vi "Encoder Reset.vi"(11 "Name of Encoder":string) -> ()   [LabVIEW 2016]
uses:
  Robot Global Data.vi
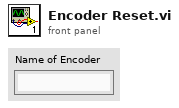
[diagram p1: front panel]
types:
  T1 = typedef "WPI_MotorControlDeviceRef.ctl" = cluster{"DeviceStatus":errorcluster, "Type":T2, "PWM":cluster{"PWM Channel":T3, "DeadBand":T4}, "CAN":cluster{"Device Number":u8, "SetOutput VI Ref":variant, "GetOutput VI Ref":variant, "Enable VI Ref":variant, "Disable VI Ref":variant, "Data":variant}, "Invert":bool}
  T2 = typedef "WPI_MotorControlType.ctl" = enum16{"PWM", "CAN"}
  T3 = typedef "FPGA_DIOPWMChannel.ctl" = enum8{"PWM 0", "PWM 1", "PWM 2", "PWM 3", "PWM 4", "PWM 5", "PWM 6", "PWM 7", "PWM 8", "PWM 9", "PWM MXP 0", "PWM MXP 1", "PWM MXP 2", "PWM MXP 3", "PWM MXP 4", "PWM MXP 5", "PWM MXP 6", "PWM MXP 7", "PWM MXP 8", "PWM MXP 9", "Invalid"}
  T4 = typedef "WPI_PWMDeadband.ctl" = cluster{"Name":string, "maxPositivePwm":i32, "minPositivePwm":i32, "centerPwm":i32, "maxNegativePwm":i32, "minNegativePwm":i32, "angularRange":u16}
  T5 = typedef "WPI_CANTalonSRX_GlobalStatus.ctl" = cluster{"Applied Throttle":dbl, "Module Enabled":bool, "CAN Error":errorcluster, "Closed Loop Error":dbl, "Forward Limit Switch Closed":bool, "Reverse Limit Switch Closed":bool, "Sensor Position":dbl, "Sensor Velocity":dbl, "Current":dbl, "Sticky Fault - Over Temp":bool, "Sticky Fault - Under Voltage":bool, "Sticky Fault - Forward Limit":bool, "Sticky Fault - Reverse Limit":bool, "Sticky Fault - Forward Soft Limit":bool, "Sticky Fault - Reverse Soft Limit":bool, "Brake is Enabled":bool, "Encoder Position":dbl, "Encoder Velocity":dbl, "Encoder Index Count":dbl, "Encoder A Pin State":bool, "Encoder B Pin State":bool, "Encoder Index Pin State":bool, "Analog In":dbl, "Analog In Velocity":dbl, "Temperature (C)":dbl, "Battery Voltage":dbl, "Control 5 Is Supported":bool, "Current Profile Slot Select":dbl, "Pos Div 8":bool, "Vel Div 4":bool, "Pulse Width Position":i32, "Pulse Width Velocity":i32, "Pulse Width Rise To Rise (us)":i32, "Pulse Width Rise To Fall (us)":i32, "Mot Prof Active Is Under Run":bool, "Mot Prof Active Has Under Run":bool, "Mot Prof Active Is Last":bool, "Mot Prof Active Velocity Only":bool, "Mot Prof Active Is Valid":bool, "Mot Prof Buffer Is Full":bool, "Mot Prof Active Profile Slot Select":i32, "Mot Prof NextID":i32, "Mot Prof Count":i32, "Mot Prof Active Velocity":dbl, "Mot Prof Active Position":dbl, "Mot Prof Output Enable":i32}
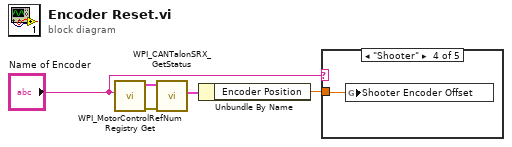
[diagram p0: block diagram]
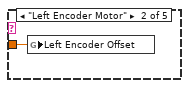
[diagram p3: hidden frame]
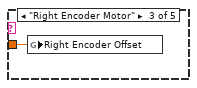
[diagram p4: hidden frame]
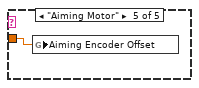
[diagram p5: hidden frame]
diagram:
  n1 = call <vilib>:"WPI_MotorControlRefNum Registry Get.vi"("refnum name"="Name of Encoder") -> ("error out"=w4:errorcluster, "MotorControlDevRef"=w3:T1)  [unwired: 9 in]
  n2 = call <vilib>:"WPI_CANTalonSRX_GetStatus.vi"("error in (no error)"=w4, "CAN Talon SRX Ref"=w3) -> ("Talon SRX Status"=w5:T5)  [unwired: 7 in, 2 out]
  n3 = Unbundle By Name(w5) -> ("Encoder Position"=w1:dbl)
  n4 = case shown="\"Shooter\"" "Name of Encoder" {
    tunnel: w1 -> [_ w6 w7 w8 w9]
    frame Default {
    }
    frame "Left Encoder Motor" {
      n5 = global write "Robot Global Data.vi" "Left Encoder Offset"(w6) -> ()
    }
    frame "Right Encoder Motor" {
      n6 = global write "Robot Global Data.vi" "Right Encoder Offset"(w7) -> ()
    }
    frame "Shooter" {
      n7 = global write "Robot Global Data.vi" "Shooter Encoder Offset"(w8) -> ()
    }
    frame "Aiming Motor" {
      n8 = global write "Robot Global Data.vi" "Aiming Encoder Offset"(w9) -> ()
    }
  }
